vi "Lockin_sweep.vi"(8 "error in (no error)":errorcluster, 10 "Configure Sweep":T2 {"Channels"."Table" format="%#_1f"; "Channels"."Channel" min=1 max=128; "Channels"."Start" format="%#_6p"; "Channels"."End" format="%#_6p"}, 11 "Transport":refnum<class "SMO.Transport.lvclass">) -> (0 "error out":errorcluster, 3 "Transport out":refnum<class "SMO.Transport.lvclass">)   [LabVIEW 2019, in "SMO.Transport.lvclass"]
uses:
  SMO.Transport.lvclass
  <userlib>/LevyLab/Instrument Framework/Instrument Types/Cryostat/Instrument.Cryostat.lvclass
  Control Experiment/Control Experiment.lvclass
  <userlib>/LevyLab/Krohn Hite 7008/Instrument.KH7008.lvclass
  <userlib>/LevyLab/Lockin-Multichannel/Instrument.Lockin/Instrument.Lockin.lvclass
  Control Experiment/Typedefs/Instruments--cluster.ctl
  <userlib>/LevyLab/Instrument Framework/Instrument Types/VSource/Instrument.VSource.lvclass
  <userlib>/LevyLab/Instrument Framework/Instrument Types/VNA/Instrument.VNA.lvclass
  <userlib>/LevyLab/Instrument Framework/Instrument Types/Strain/Instrument.Strain.lvclass
  <userlib>/LevyLab/Instrument Framework/Instrument Types/CBridge/Instrument.CBridge.lvclass
  <userlib>/LevyLab/Lockin-Multichannel/Instrument.DAQ/Typedefs/Sweep.Configuration--Cluster.ctl
  <userlib>/LevyLab/Lockin-Multichannel/Instrument.DAQ/Instrument.DAQ.lvclass
  <userlib>/LevyLab/Lockin-Multichannel/Instrument.DAQ/Typedefs/Set State-enum.ctl
  <userlib>/_OpenG.lib/array/array.llb/Index 1D Array Elements (Variant)__ogtk.vi
  <userlib>/LevyLab/Lockin-Multichannel/Instrument.Lockin/Typedefs/Results Type--Enum.ctl
  <userlib>/LevyLab/Instrument Framework/Instrument Types/Delay Line/Instrument.DelayLine.lvclass
  <userlib>/LevyLab/Lockin-Multichannel/Instrument.DAQ/Typedefs/Sweep.Pattern--Enum.ctl
  <userlib>/LevyLab/Lockin-Multichannel/Instrument.DAQ/Typedefs/Sweep.Channel--Cluster.ctl
  <userlib>/LevyLab/Lockin-Multichannel/Instrument.DAQ/Typedefs/Sweep.Channel--Cluster--Array.ctl
  SMO.Control Experiment/SMO.Control Experiment.lvclass
  C:/Program Files (x86)/National Instruments/LabVIEW 2019/user.lib/LevyLab/Instrument Framework/SMOs/Instrument/Instrument.lvclass
  C:/Program Files (x86)/National Instruments/LabVIEW 2019/vi.lib/JKI/JKI SMO/SMO/SMO.lvclass
panel:
  in  "Tab Control":T1(tab)
  out "elapsed time (s)":u32=231
  in  "Experiment Comments":string="sweep inplane y gates in differential mode, 110Mohm resistor on each\nlead 3: +X: 0 V\nlead 15: -X: 0V\nlead 8: +Y: -10V to 10V to -10V to 10V...\nlead 21: -Y: 10V to -10V to 10V to -10V..\n\nInital wait: 2s+ 2s\nSweep Time: 90s+90s\n\nstripe device\nI+: 11,12, current mode, 5k resistor on each, 1000x gain\nlead 12: Vac: 125uV, 7Hz. Vdc=0mV\ndV: KH channel 16: 11-12, differential voltage meas, 10x gain \n\nhash device\nI+: 16,27, current mode, 5k resistor on each, 1000x gain\nlead 16: Vac: 5mV, 7Hz. Vdc=0mV\nV+/V-: 17/20, voltage meas, 10x gain \nKH 5: 17-20, volt. meas., 10x gain\n\n\nlead 26: Vbg: 0V, 1Gohm resistor\nB: -18T to 18T @0.033T/min\n"
  in  "Experiment Folder":string="23-Lockinsweep_ygates_-18_18"
  out "T (mK)":dbl=0.001
  out "Field (T)":dbl=0.0037 format="%#_13g"
  out "time b/w points (ms)":u32=1037
  in  "stop":bool
  out "X Lockins":cluster{dbl[], dbl[]}[](graph)
  out "Y Lockins":cluster{dbl[], dbl[]}[](graph)
  out "G4T":cluster{dbl[], dbl[]}[](graph)
  out "AI Waveform":waveform(dbl)[](graph)
  out "AO Waveform":waveform(dbl)[](graph)
  in  "AO indices":i32[](array[numeric])
  in  "AI indices":i32[](array[numeric])
  out "2Term":T6(graph)
  out "4Term":cluster{dbl[], dbl[]}[](graph)
  # "VI description:\nThis VI uses the Lockin Sweep Method. That is, you tell the lockin to sweep from Start to End in a certain amount of time. The lockin will run independently while it executes the sweep. While the lockin is sweeping, this VI will poll the lockin once per second to get a snapshot of current results and the sweep status (sweeping or not sweeping). When the lockin is finished sweeping this VI will ask for the final sweep results and save them."
  # "*** These controls are only read if this VI is the top level. If is is called from Sweep Control then the folder and comments come from Sweep Control.vi ***"
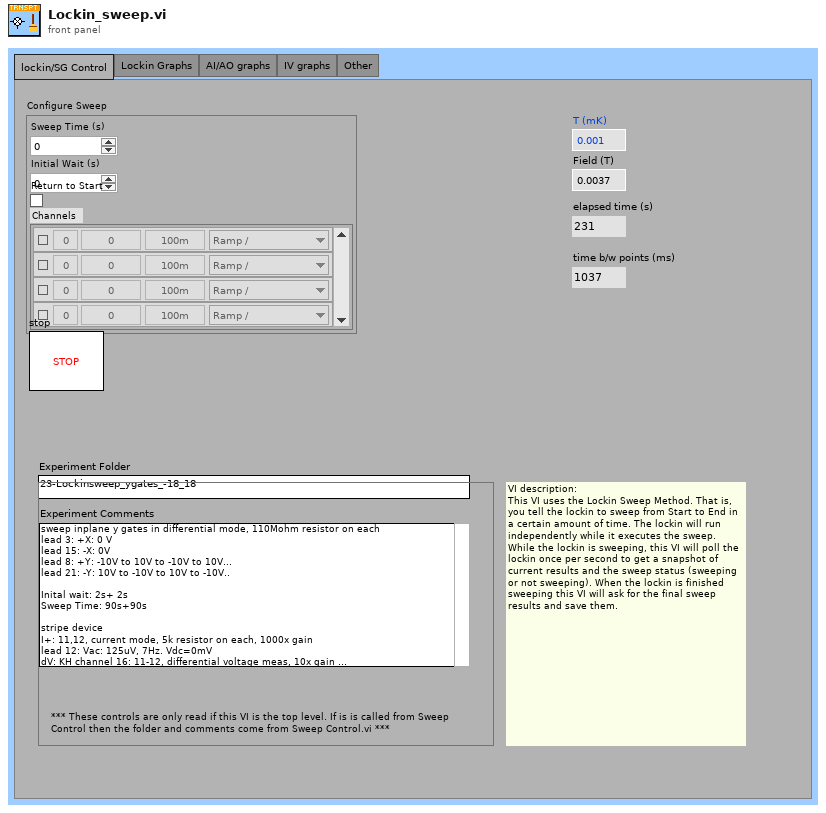
[diagram p1: front panel]
types:
  T1 = enum32{"lockin/SG Control", "Lockin Graphs", "AI/AO graphs", "IV graphs", "Other"}
  T2 = typedef "Instrument.DAQ.lvclass/Sweep.Configuration--Cluster.ctl" = cluster{"Sweep Time (s)":dbl, "Initial Wait (s)":dbl, "Return to Start":bool, "Channels":T3}
  T3 = typedef "Instrument.DAQ.lvclass/Sweep.Channel--Cluster--Array.ctl" = T4[]
  T4 = typedef "Instrument.DAQ.lvclass/Sweep.Channel--Cluster.ctl" = cluster{"Enable?":bool, "Channel":u16, "Start":dbl, "End":dbl, "Pattern":T5, "Table":dbl[]}
  T5 = typedef "Instrument.DAQ.lvclass/Sweep.Pattern--Enum.ctl" = enum16{"Ramp /", "Ramp /\\", "Smooth Ramp _/", "Smooth Ramp _/\\_", "Table"}
  T6 = cluster{"Decimated and Filtered Array":dbl[], "Decimated and Filtered Array":dbl[]}[]
  T7 = enum32{"Invalid", "Standard", "Closed", "Hidden", "Minimized", "Maximized"}
  T8 = enum32{"invalid app kind", "Development System", "Run Time System", "Student Edition", "Embedded LabVIEW", "Evaluation", "Custom"}
  T9 = typedef "Instrument.Lockin.lvclass/Results Type--Enum.ctl" = enum16{"X", "Y", "R", "Theta", "Mean"}
  T10 = typedef "Lockin.DAQ.lvclass/State-enum.ctl" = enum16{"idle", "created", "started", "stopped", "sweeping"}
  T11 = typedef "Control Experiment.lvclass/Instruments--cluster.ctl" = cluster{"KH7008":refnum<class "Instrument.KH7008.lvclass">[], "Lockin":refnum<class "Instrument.Lockin.lvclass">, "Temperature":refnum<class "Instrument.Cryostat.lvclass">, "Magnet":refnum<class "Instrument.Cryostat.lvclass">, "Rotator":refnum<class "Instrument.Cryostat.lvclass">, "Level":refnum<class "Instrument.Cryostat.lvclass">, "Capacitance Bridge":refnum<class "Instrument.CBridge.lvclass">, "Delay Line":refnum<class "Instrument.DelayLine.lvclass">, "Strain Cell":refnum<class "Instrument.Strain.lvclass">, "VNA":refnum<class "Instrument.VNA.lvclass">, "Voltage Source":refnum<class "Instrument.VSource.lvclass">}
  T12 = cluster{"Core":cluster{"Current VI Reference":refnum<vi>, "Close Panel on Exit?":bool}, "Transport":refnum<class "SMO.Transport.lvclass">, "Control Experiment":refnum<class "SMO.Control Experiment.lvclass">, "Instruments":T11, "Time":dbl, "Temperature":dbl, "Magnet":dbl, "Results (Dictionary)":cluster{"key":string, "value":dbl}[], "Sweep Value":dbl, "ms [0]":u32, "ms [i]":u32, "Execution:State":enum32{"Bad", "Idle", "Run top level", "Running"}, "AO Waveforrm":waveform(dbl)[], "AI Waveform":waveform(dbl)[], "Sweep_AO":waveform(dbl)[], "Sweep_AI":waveform(dbl)[]}
  T13 = enum32{"Bad", "Idle", "Run top level", "Running"}
  T14 = cluster{"Current VI Reference":refnum<vi>, "Close Panel on Exit?":bool}
  T15 = cluster{"I-":i32, "I+":i32, "V1-":i32, "V1+":i32, "I2-":i32, "I2+":i32, "V2-":i32, "V2+":i32}
  T16 = typedef "Instrument.DAQ.lvclass/Get State-enum.ctl" = enum16{"idle", "created", "started", "stopped", "sweeping"}
  T17 = typedef "Instrument.DAQ.lvclass/AO.Channel--Cluster--Array.ctl" = T18[]
  T18 = typedef "Instrument.DAQ.lvclass/AO.Channel--Cluster.ctl" = cluster{"Enable?":bool, "Channel":i32, "Amplitude":dbl, "Offset":dbl, "Frequency":dbl, "Phase":dbl, "Function":T19, "Sweeping?":bool}
  T19 = typedef "Instrument.DAQ.lvclass/AO.Channel.Function--Enum.ctl" = enum16{"Sine", "Triangle", "Square"}
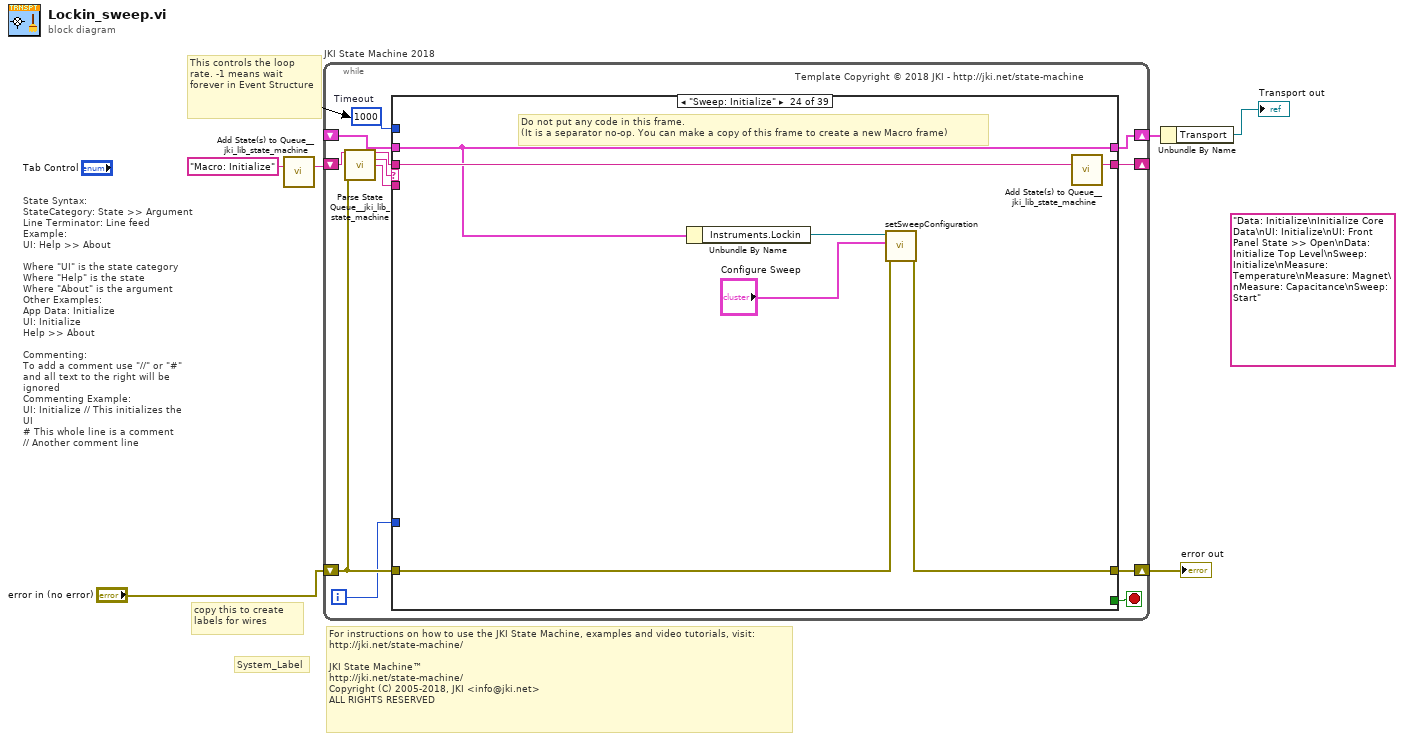
[diagram p0: block diagram]
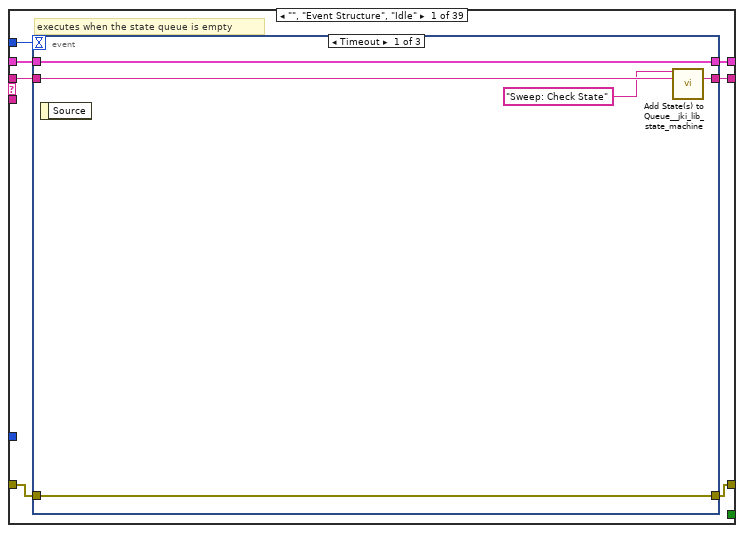
[diagram p2: hidden frame]
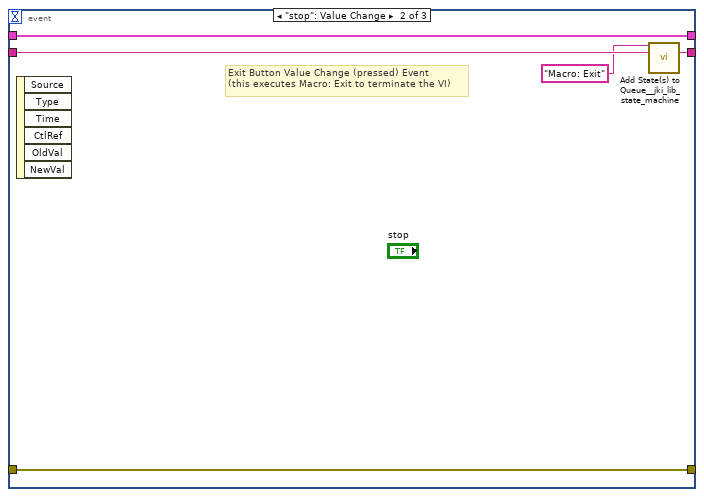
[diagram p3: hidden frame]
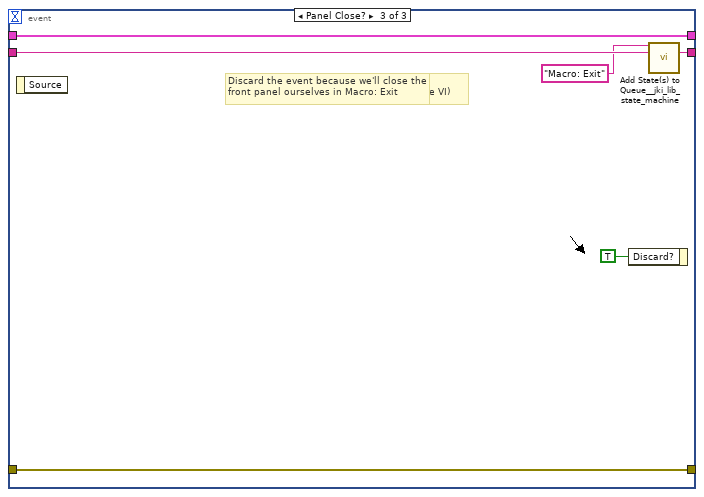
[diagram p4: hidden frame]
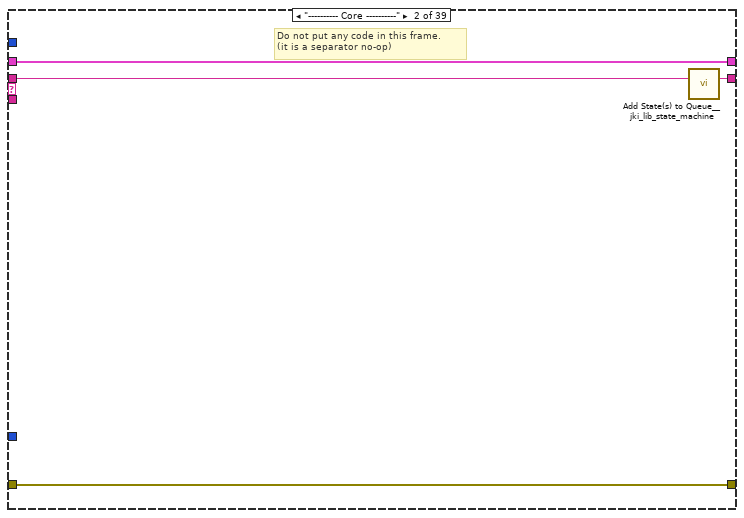
[diagram p5: hidden frame]
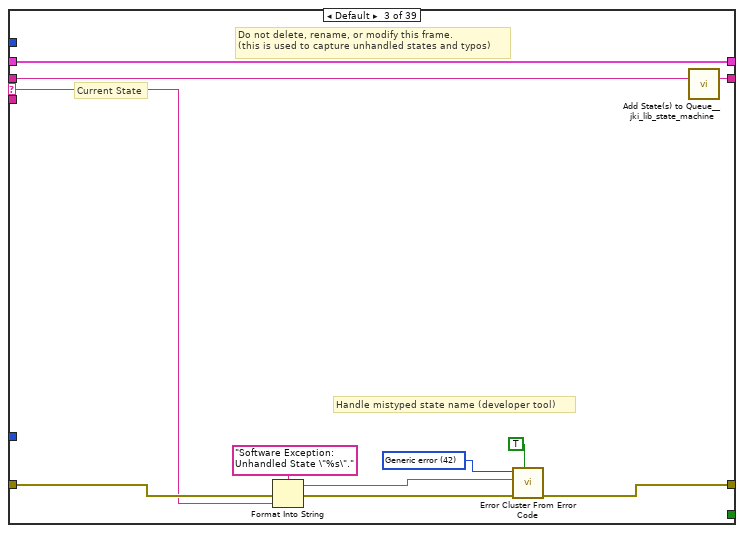
[diagram p6: hidden frame]
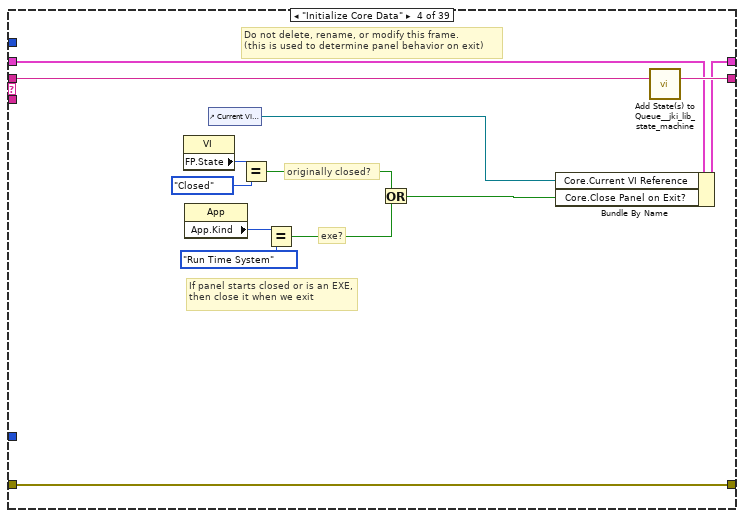
[diagram p7: hidden frame]
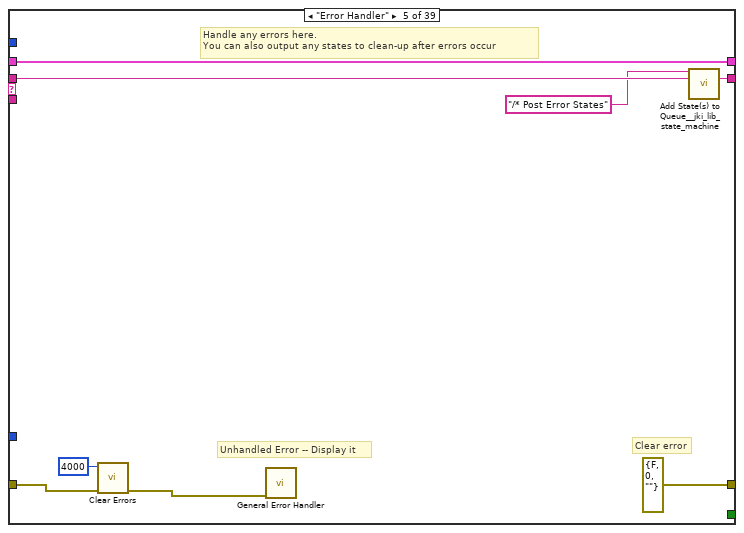
[diagram p8: hidden frame]
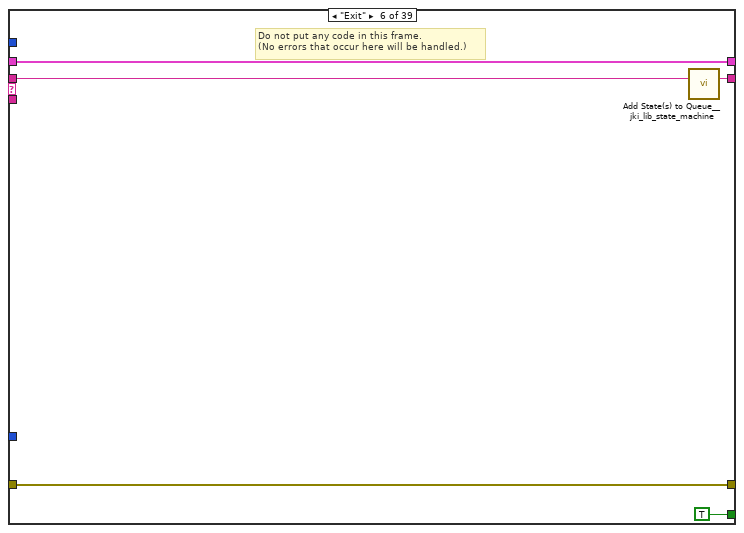
[diagram p9: hidden frame]
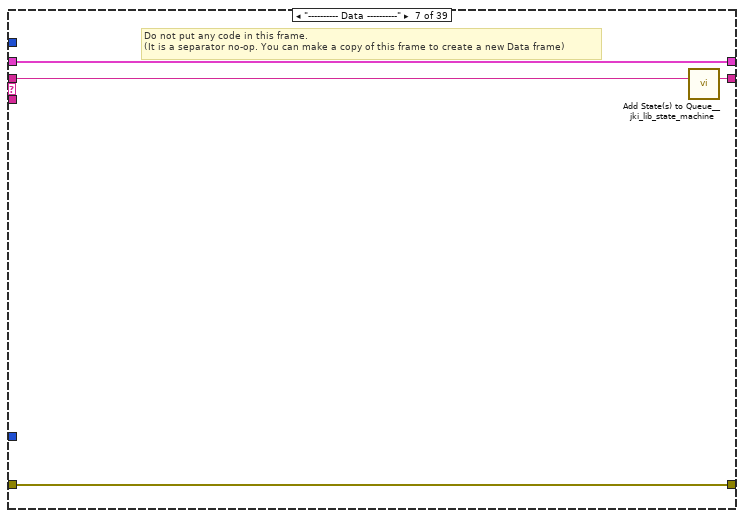
[diagram p10: hidden frame]
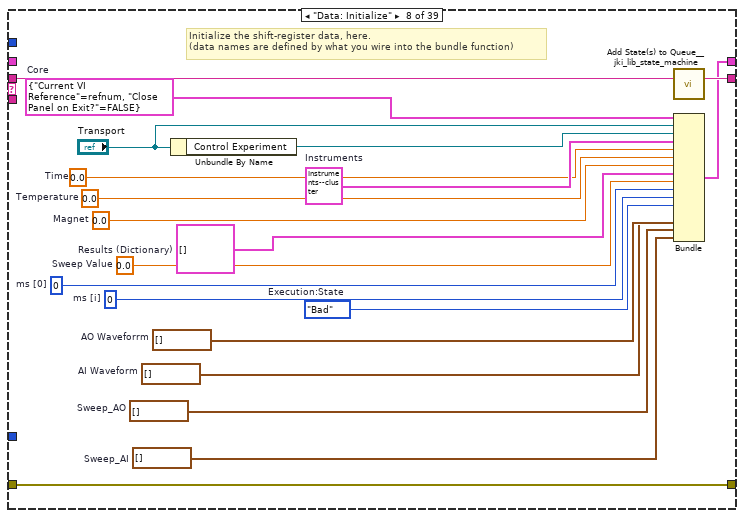
[diagram p11: hidden frame]
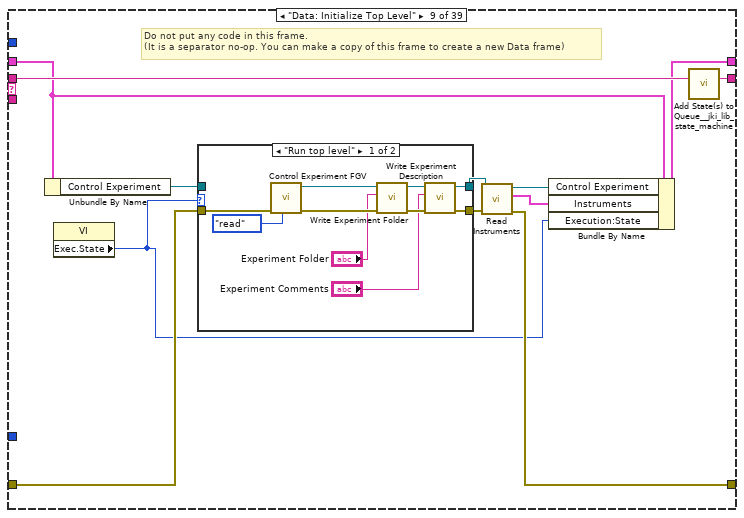
[diagram p12: hidden frame]
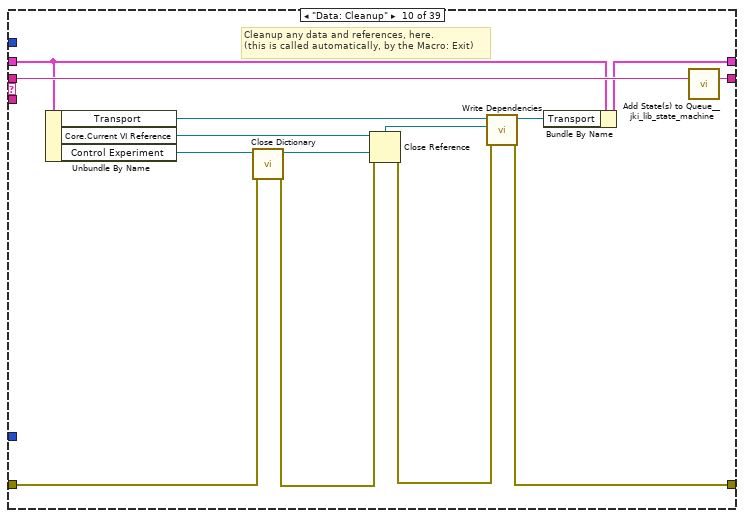
[diagram p14: hidden frame]
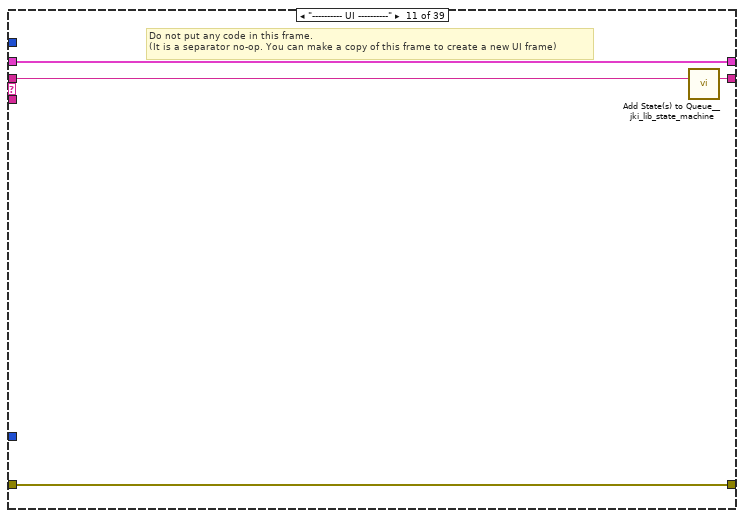
[diagram p15: hidden frame]
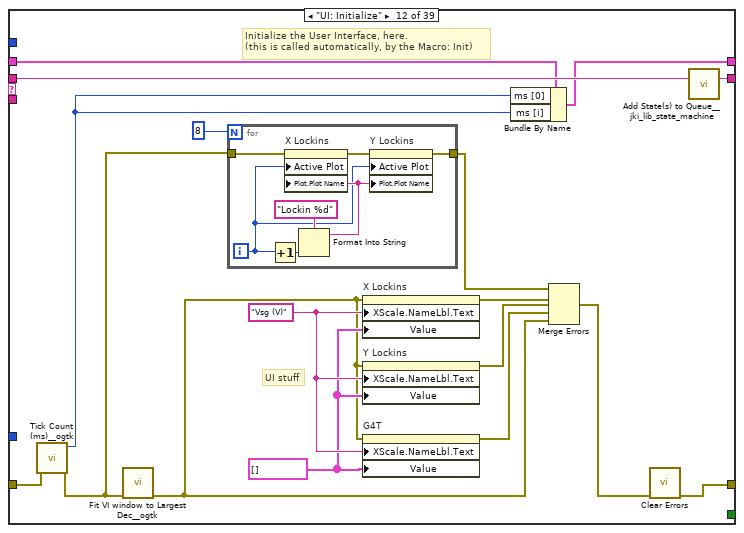
[diagram p16: hidden frame]
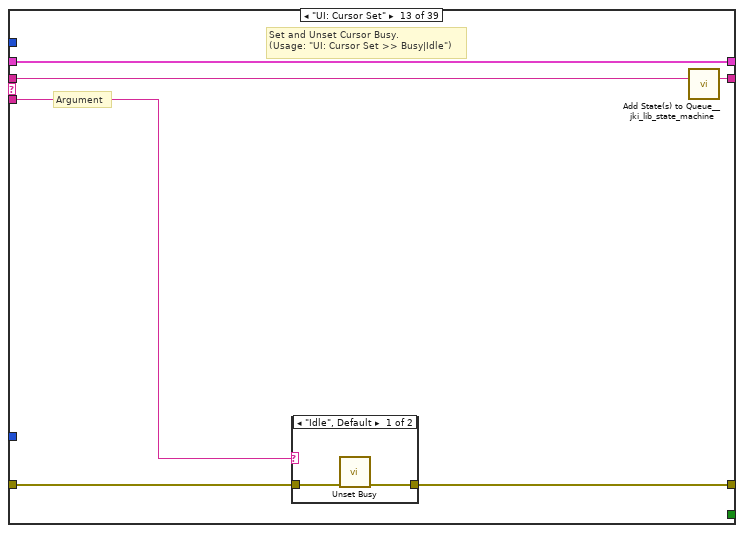
[diagram p17: hidden frame]
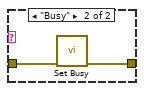
[diagram p18: hidden frame]
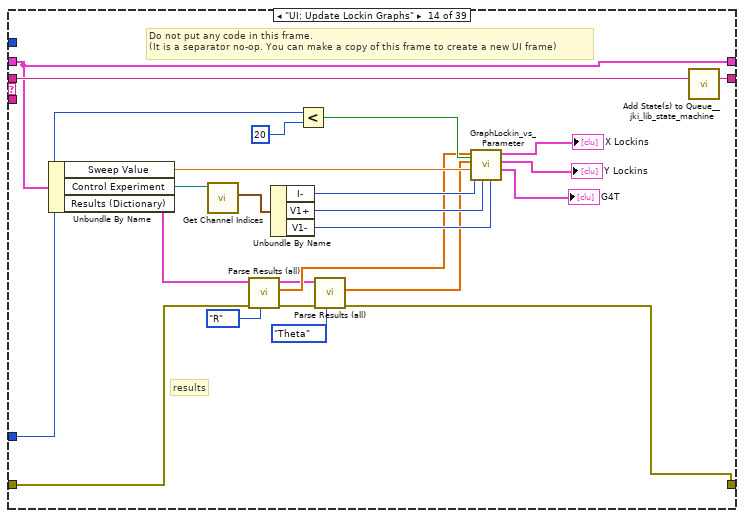
[diagram p19: hidden frame]
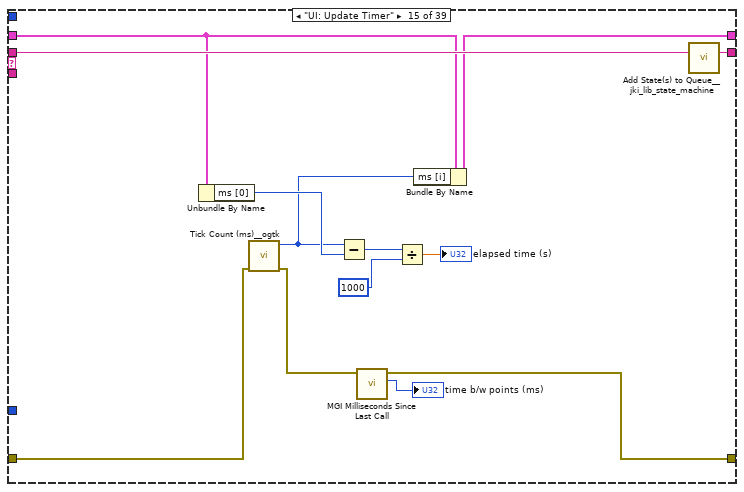
[diagram p20: hidden frame]
diagram:
  (unwired) "Data: Initialize\nInitialize Core Data\nUI: Initialize\nUI: Front Panel State >> Open\nData: Initialize Top Level\nSweep: Initialize\nMeasure: Temperature\nMeasure: Magnet\nMeasure: Capacitance\nSweep: Start"
  # "For instructions on how to use the JKI State Machine, examples and video tutorials, visit:\nhttp://jki.net/state-machine/\n\nJKI State Machine™\nhttp://jki.net/state-machine/\nCopyright (C) 2005-2018, JKI <info@jki.net>\nALL RIGHTS RESERVED"
  # "State Syntax:\nStateCategory: State >> Argument\nLine Terminator: Line feed\nExample:\nUI: Help >> About\n\nWhere \"UI\" is the state category\nWhere \"Help\" is the state\nWhere \"About\" is the argument\nOther Examples:\nApp Data: Initialize\nUI: Initialize\nHelp >> About\n\nCommenting:\nTo add a comment use \"//\" or \"#\" and all text to the right will be ignored\nCommenting Example:\nUI: Initialize // This initializes the UI\n# This whole line is a comment\n// Another comment line"
  # "copy this to create labels for wires"
  # "This controls the loop rate. -1 means wait forever in Event Structure"
  # "System_Label"
  n1 = call <vilib>:"Add State(s) to Queue__jki_lib_state_machine.vi"("State(s) in (\"\")"="Macro: Initialize") -> ("States Out"=w6:string)  [unwired: 14 in]
  n2 = while "JKI State Machine 2018" {
    shift-right: [w11] -> w4
    shift-left: _ -> [w10]
    shift-right: [w14] -> w2
    shift-left: "error in (no error)" -> [w8]
    shift-right: [w13] -> _
    shift-left: w6 -> [w15]
    i -> [w7]
    stop <- w12 stop-if-true
    w9 = 1000  # Timeout
    # "Template Copyright © 2018 JKI - http://jki.net/state-machine"
    n3 = call <vilib>:"Parse State Queue__jki_lib_state_machine.vi"("State Queue"=w15, "Error In (no error)"=w8) -> ("Remaining States"=w17:string, "Current State"=w18:string, "Arguments"=w16:string)  [unwired: 11 in]
    n4 = case shown="\"Sweep: Initialize\"" w18 {
      selector: w18 -> [_ _ w46 _ _ _ _ _ _ _ _ _ _ _ _ _ _ _ _ _ _ _ _ _ _ _ _ _ _ _ _ _ _ _ _ _ _ _ _]
      tunnel: w17 -> [w25 w45 w50 w69 w77 w82 w86 w106 w118 w143 w147 w164 w177 w205 w218 w232 w263 w270 w339 w344 w349 w359 w363 w370 w378 w393 w401 w407 w411 w415 w426 w439 w452 w464 w486 w490 w494 w527 w546]
      tunnel: w16 -> [_ _ _ _ _ _ _ _ _ _ _ _ w172 _ _ _ _ w264 _ _ _ _ _ _ _ _ _ _ _ _ _ _ _ _ _ _ _ _ _]
      tunnel: w10 -> [w23 w42 w48 w62 w74 w80 w83 _ w109 w131 w144 w152 w175 w202 w213 w222 w242 w266 w336 w342 w345 w356 w360 w365 w376 w391 w399 w404 w409 w412 w422 w435 w450 w453 w465 w487 w491 w516 w543]
      tunnel: [w22 w43 w52 w66 errorcluster {"status"=FALSE, "code"=0, "source"=""} ("error out") w79 w84 w103 w110 w133 w145 w156 w173 w182 w207 w230 w240 w267 w337 w340 w347 w357 w361 w366 w371 w388 w396 w405 w408 w413 w416 w428 w446 w459 w484 w488 w492 w519 w541] -> w14
      tunnel: w8 -> [w21 w43 w51 w66 w71 w79 w84 w103 w111 w139 w145 w154 w174 w184 w215 w230 w241 w268 w337 w340 w347 w357 w361 w367 w374 w389 w397 w405 w408 w413 w417 w436 w443 w457 w482 w488 w492 w498 w542]
      tunnel: [w24 w44 w49 w68 w76 w81 w85 w105 w117 w142 w146 w163 w176 w204 w217 w231 w262 w269 w338 w343 w348 w358 w362 w369 w377 w392 w400 w406 w410 w414 w425 w438 w451 w463 w485 w489 w493 w526 w545] -> w13
      tunnel: [_ _ _ _ _ TRUE _ _ _ _ _ _ _ _ _ _ _ _ _ _ _ _ _ _ _ _ _ _ _ _ _ _ _ _ _ _ _ _ _] -> w12
      tunnel: [w20 w42 w48 w67 w74 w80 w83 w104 w108 w135 w144 w151 w175 w202 w212 w221 w242 w266 w336 w342 w345 w356 w360 w365 w376 w391 w399 w404 w409 w412 w423 w434 w449 w462 w466 w487 w491 w515 w543] -> w11
      tunnel: w9 -> [w19 _ _ _ _ _ _ _ _ _ _ _ _ _ _ _ _ _ _ _ _ _ _ _ _ _ _ _ _ _ _ _ _ _ _ _ _ _ _]
      tunnel: w7 -> [_ _ _ _ _ _ _ _ _ _ _ _ _ w193 _ _ _ _ _ _ _ _ _ _ _ _ _ _ _ _ _ _ _ _ _ _ _ _ _]
      frame "", "Event Structure", "Idle" {
        # "executes when the state queue is empty"
        n5 = event shown="[0] Timeout" {
          selector: _ -> [_ _ _]
          dyn-events: _ -> [_ _ _]
          timeout: w19 -> [_ _ _]
          tunnel: w25 -> [w30 w35 w41]
          tunnel: [w29 w34 w40] -> w24
          tunnel: w23 -> [w27 w32 w38]
          tunnel: [w28 w33 w39] -> w22
          tunnel: w21 -> [w28 w33 w39]
          tunnel: [w27 w32 w38] -> w20
          event Timeout {
            n6 = event-data() -> ()  [unwired: 1 in, 1 out]
            n7 = call <vilib>:"Add State(s) to Queue__jki_lib_state_machine.vi"("State(s) in Front (\"\")"="Sweep: Check State" ("State(s) in Front (\"\")"), "State(s) in (\"\")"=w30) -> ("States Out"=w29:string)  [unwired: 13 in]
          }
          event "stop": Value Change {
            # "Exit Button Value Change (pressed) Event\n(this executes Macro: Exit to terminate the VI)"
            n8 = event-data() -> ()  [unwired: 1 in, 6 out]
            n9 = call <vilib>:"Add State(s) to Queue__jki_lib_state_machine.vi"("State(s) in Front (\"\")"="Macro: Exit", "State(s) in (\"\")"=w35) -> ("States Out"=w34:string)  [unwired: 13 in]
          }
          event Panel Close? {
            # "Discard the event because we'll close the front panel ourselves in Macro: Exit"
            # "Close Panel button (pressed) Event\n(this executes Macro: Exit to terminate the VI)"
            n10 = event-data() -> ()  [unwired: 1 in, 1 out]
            n11 = event-data("Discard?"=TRUE) -> ()  [unwired: 1 in, 1 out]
            n12 = call <vilib>:"Add State(s) to Queue__jki_lib_state_machine.vi"("State(s) in Front (\"\")"="Macro: Exit", "State(s) in (\"\")"=w41) -> ("States Out"=w40:string)  [unwired: 13 in]
          }
        }
      }
      frame "---------- Core ----------" {
        # "Do not put any code in this frame.\n(it is a separator no-op)"
        n13 = call <vilib>:"Add State(s) to Queue__jki_lib_state_machine.vi"("State(s) in (\"\")"=w45) -> ("States Out"=w44:string)  [unwired: 14 in]
      }
      frame Default {
        w55 = 42 items=["No error", "Argument error", "Memory is full", "Out of zone", "End of file", "File already open", "Generic file I/O error", "File not found", "File permission error", "Disk is full", "Duplicate path", "Too many files open", "System feature not enabled", "Resource file not found", "Cannot add resource", "Resource not found", "Image not found", "Image memory error", "Pen does not exist", "Config type invalid", "Config token not found", "Config parse error", "Config memory error", "Bad external code format", "Bad external code offset", "External code not present", "Null window", "Destroy window error", "Null menu", "Print aborted", "Bad print record", "Print driver error", "Windows error during printing", "Memory error during printing", "Print dialog error", "Generic print error", "Invalid device refnum", "Device not found", "Device parameter error", "Device unit error", "Cannot open device", "Device call aborted", "Generic error", "Cancelled by user", "Object ID too low", "Object ID too high", "Object not in heap", "Unknown heap", "Unknown object (invalid DefProc)", "Unknown object (DefProc not in table)", "Message out of range", "Invalid (null) method", "Unknown message", "Manager call not supported", "Bad address", "Network operation in progress", "Network operation timed out", "Connection is busy", "Network attribute not supported", "Network error", "Address in use", "System out of memory", "Connection aborted", "Connection refused", "Not connected", "Already connected", "Connection closed", "Initialization error (interapplication manager)", "Bad occurrence", "Wait on unbound occurrence handler", "Occurrence queue overflow", "Datalog type conflict", "Unused", "Unrecognized type (interapplication manager)", "Memory corrupt", "Failed to make temporary DLL", "Old CIN version", "Drag socket not found", "Failed to load drop-object", "Failed to register OLE object", "Failed to release OLE object", "Format specifier type mismatch", "Unknown format specifier", "Too few format specifiers", "Too many format specifiers", "Scan failed", "Newer CIN version", "Error converting to variant", "Runtime menu error", "Password tampered", "Variant attribute not found", "Incompatible variant data type", "Event data is not available", "Event Store is not present", "Occurrence is not found", "Event Queue is not created", "Event info is not available", "Refnum passed is NULL", "Error retrieving Class GUID", "Error retrieving CoClass GUID", "Error retrieving TypeLib GUID.", "Bad built application magic bytes.", "Specific driver is different from the specific driver associated with the Logical Name.", "There is no session opened to the class driver.", "Max Error", "MAX - Error with config objects", "MAX - Error loading configuration", "MAX - Group not supported"]
        # "Current State"
        # "Do not delete, rename, or modify this frame.\n(this is used to capture unhandled states and typos)"
        # "Handle mistyped state name (developer tool)"
        n14 = Format Into String(format string="Software Exception: Unhandled State \"%s\"." ("message"), error in=w51, w46) -> (resulting string=w54:string, error out=w53:errorcluster)  [unwired: 1 in]
        n15 = call <vilib>:"Error Cluster From Error Code.vi"("show call chain? (False)"=TRUE, "error in (no error)"=w53, "error message (\"\")"=w54, "error code (0)"=w55) -> ("error out"=w52:errorcluster)  [unwired: 5 in]
        n16 = call <vilib>:"Add State(s) to Queue__jki_lib_state_machine.vi"("State(s) in (\"\")"=w50) -> ("States Out"=w49:string)  [unwired: 14 in]
      }
      frame "Initialize Core Data" {
        # "Do not delete, rename, or modify this frame.\n(this is used to determine panel behavior on exit)"
        # "originally closed?"
        # "exe?"
        # "If panel starts closed or is an EXE, then close it when we exit"
        n17 = property class="VI"() -> ("FP.State"=w59:T7)  [unwired: 2 in, 2 out]
        n18 = property class="App"() -> ("App.Kind"=w65:T8)  [unwired: 2 in, 2 out]
        n19 = control-ref of="Current VI Reference"() -> (w60:refnum<vi>)
        n20 = Equal?(x=w59, y=T7."Closed" ("Front Panel Window:State")) -> (x = y?=w57:bool)
        n21 = Equal?(x=w65, y=T8."Run Time System" ("Application:Kind")) -> (x = y?=w63:bool)
        n22 = Or(x=w57, y=w63) -> (x .or. y?=w61:bool)
        n23 = Bundle By Name(cluster=w62, "Core.Current VI Reference"=w60, "Core.Close Panel on Exit?"=w61) -> (w67:T12)
        n24 = call <vilib>:"Add State(s) to Queue__jki_lib_state_machine.vi"("State(s) in (\"\")"=w69) -> ("States Out"=w68:string)  [unwired: 14 in]
      }
      frame "Error Handler" {
        # "Unhandled Error -- Display it"
        # "Handle any errors here.\nYou can also output any states to clean-up after errors occur"
        # "Clear error"
        n25 = call <vilib>:"Clear Errors.vi"("error in (no error)"=w71, "specific error code to clear (0: all)"=4000) -> ("error out"=w70:errorcluster)  [unwired: 4 in, 1 out]
        n26 = call <vilib>:"General Error Handler.vi"("error in (no error)"=w70) -> ()  [unwired: 10 in, 5 out]
        n27 = call <vilib>:"Add State(s) to Queue__jki_lib_state_machine.vi"("State(s) in Front (\"\")"="/* Post Error States", "State(s) in (\"\")"=w77) -> ("States Out"=w76:string)  [unwired: 13 in]
      }
      frame "Exit" {
        # "Do not put any code in this frame.\n(No errors that occur here will be handled.)"
        n28 = call <vilib>:"Add State(s) to Queue__jki_lib_state_machine.vi"("State(s) in (\"\")"=w82) -> ("States Out"=w81:string)  [unwired: 14 in]
      }
      frame "---------- Data ----------" {
        # "Do not put any code in this frame.\n(It is a separator no-op. You can make a copy of this frame to create a new Data frame)"
        n29 = call <vilib>:"Add State(s) to Queue__jki_lib_state_machine.vi"("State(s) in (\"\")"=w86) -> ("States Out"=w85:string)  [unwired: 14 in]
      }
      frame "Data: Initialize" {
        w87 = cluster{"key":string, "value":dbl}[] []  # Results (Dictionary)
        w89 = waveform(dbl)[] []  # Sweep_AO
        w88 = waveform(dbl)[] []  # Sweep_AI
        w90 = waveform(dbl)[] []  # AI Waveform
        w91 = waveform(dbl)[] []  # AO Waveforrm
        w92 = T13."Bad"  # Execution:State
        w93 = 0.0  # Sweep Value
        w95 = u32 0  # ms [i]
        w96 = u32 0  # ms [0]
        w98 = 0.0  # Time
        w99 = 0.0  # Magnet
        w97 = 0.0  # Temperature
        w100 = T11 {"KH7008"=[], "Lockin"=refnum, "Temperature"=refnum, "Magnet"=refnum, "Rotator"=refnum, "Level"=refnum, "Capacitance Bridge"=refnum, "Delay Line"=refnum, "Strain Cell"=refnum, "VNA"=refnum, "Voltage Source"=refnum}  # Instruments
        w102 = T14 {"Current VI Reference"=refnum, "Close Panel on Exit?"=FALSE}  # Core
        # "Initialize the shift-register data, here.\n(data names are defined by what you wire into the bundle function)"
        n30 = Unbundle By Name("Transport") -> ("Control Experiment"=w94:refnum<class "SMO.Control Experiment.lvclass">)
        n31 = call <vilib>:"Add State(s) to Queue__jki_lib_state_machine.vi"("State(s) in (\"\")"=w106) -> ("States Out"=w105:string)  [unwired: 14 in]
        n32 = Bundle("Core"=w102, "Transport"="Transport", "Control Experiment"=w94, "Instruments"=w100, "Time"=w98, "Temperature"=w97, "Magnet"=w99, "Results (Dictionary)"=w87, "Sweep Value"=w93, "ms [0]"=w96, "ms [i]"=w95, "Execution:State"=w92, "AO Waveforrm"=w91, "AI Waveform"=w90, "Sweep_AO"=w89, "Sweep_AI"=w88) -> (w104:T12)  [unwired: 1 in]
      }
      frame "Data: Initialize Top Level" {
        # "Do not put any code in this frame.\n(It is a separator no-op. You can make a copy of this frame to create a new Data frame)"
        n33 = Unbundle By Name(w109) -> ("Control Experiment"=w112:refnum<class "SMO.Control Experiment.lvclass">)
        n34 = property class="VI"() -> ("Exec.State"=w107:T13)  [unwired: 2 in, 2 out]
        n35 = case shown="\"Run top level\"" w107 {
          tunnel: w111 -> [w128 w129]
          tunnel: [w123 w129] -> w113
          tunnel: [w122 w130] -> w114
          tunnel: w112 -> [_ w130]
          frame "Run top level" {
            n36 = call "Control Experiment FGV.vi"("Function"=enum16{"read", "write"}."read", "error in (no error)"=w128) -> ("error out"=w126:errorcluster, "Control Experiment.lvclass out"=w127:refnum<class "Control Experiment.lvclass">)  [unwired: 8 in]
            n37 = call "Write Experiment Folder.vi"("error in (no error)"=w126, "Experiment Folder"="Experiment Folder", "Control Experiment in"=w127) -> ("error out"=w124:errorcluster, "Control Experiment out"=w125:refnum<class "Control Experiment.lvclass">)  [unwired: 7 in]
            n38 = call "Write Experiment Description.vi"("error in (no error)"=w124, "Experiment Description"="Experiment Comments", "Control Experiment in"=w125) -> ("error out"=w123:errorcluster, "Control Experiment out"=w122:refnum<class "Control Experiment.lvclass">)  [unwired: 7 in]
          }
          frame "Running", Default {
          }
        }
        n39 = call "Read Instruments.vi"("error in (no error)"=w113, "Control Experiment in"=w114) -> ("error out"=w110:errorcluster, "Instruments"=w116:T11, "Control Experiment out"=w115:refnum<class "Control Experiment.lvclass">)  [unwired: 7 in]
        n40 = Bundle By Name(cluster=w109, "Control Experiment"=w115, "Instruments"=w116, "Execution:State"=w107) -> (w108:T12)
        n41 = call <vilib>:"Add State(s) to Queue__jki_lib_state_machine.vi"("State(s) in (\"\")"=w118) -> ("States Out"=w117:string)  [unwired: 14 in]
      }
      frame "Data: Cleanup" {
        # "Cleanup any data and references, here.\n(this is called automatically, by the Macro: Exit)"
        n42 = Unbundle By Name(w131) -> ("Transport"=w136:refnum<class "SMO.Transport.lvclass">, "Core.Current VI Reference"=w141:refnum<vi>, "Control Experiment"=w140:refnum<class "SMO.Control Experiment.lvclass">)
        n43 = call "Close Dictionary.vi"("error in (no error)"=w139, "Control Experiment in"=w140) -> ("error out"=w138:errorcluster, "Control Experiment out"=w132:refnum<class "Control Experiment.lvclass">)  [unwired: 8 in]
        n44 = Close Reference(reference=w141, error in (no error)=w138) -> (error out=w134:errorcluster)
        n45 = call "Write Dependencies.vi"("error in (no error)"=w134, "Control Experiment"=w132, "Transport in"=w136) -> ("error out"=w133:errorcluster, "Transport out"=w137:refnum<class "SMO.Transport.lvclass">)  [unwired: 7 in]
        n46 = Bundle By Name(cluster=w131, "Transport"=w137) -> (w135:T12)
        n47 = call <vilib>:"Add State(s) to Queue__jki_lib_state_machine.vi"("State(s) in (\"\")"=w143) -> ("States Out"=w142:string)  [unwired: 14 in]
      }
      frame "---------- UI ----------" {
        # "Do not put any code in this frame.\n(It is a separator no-op. You can make a copy of this frame to create a new UI frame)"
        n48 = call <vilib>:"Add State(s) to Queue__jki_lib_state_machine.vi"("State(s) in (\"\")"=w147) -> ("States Out"=w146:string)  [unwired: 14 in]
      }
      frame "UI: Initialize" {
        w149 = cluster{dbl[], dbl[]}[] [] ("G4T")
        w158 = "Vsg (V)" ("string")
        # "UI stuff"
        # "Initialize the User Interface, here.\n(this is called automatically, by the Macro: Init)"
        n49 = call <userlib>:"Tick Count (ms)__ogtk.vi"("error in (no error)"=w154) -> ("error out"=w153:errorcluster, "millisecond timer value"=w150:u32)  [unwired: 9 in]
        n50 = call <userlib>:"Fit VI window to Largest Dec__ogtk.vi"("error in (no error)"=w153) -> ("error out"=w148:errorcluster)  [unwired: 5 in, 1 out]
        n51 = for {
          N: 8 -> [_]
          tunnel: [w165] -> w159
          tunnel: w153 -> [w170]
          i -> [w168]
          n52 = Increment(x=w168) -> (x+1=w166:i32)
          n53 = Format Into String(format string="Lockin %d", w166) -> (resulting string=w169:string)  [unwired: 2 in, 1 out]
          n54 = property on="X Lockins" class="XYGraph (strict)"(error in=w170, "Active Plot"=w168, "Plot.Plot Name"=w169) -> (error out=w167:errorcluster)  [unwired: 1 in, 1 out]
          n55 = property on="Y Lockins" class="XYGraph (strict)"(error in=w167, "Active Plot"=w168, "Plot.Plot Name"=w169) -> (error out=w165:errorcluster)  [unwired: 1 in, 1 out]
        }
        n56 = property on="X Lockins" class="XYGraph (strict)"(error in=w148, "XScale.NameLbl.Text"=w158, "Value"=w149) -> (error out=w160:errorcluster)  [unwired: 1 in, 1 out]
        n57 = property on="Y Lockins" class="XYGraph (strict)"(error in=w148, "XScale.NameLbl.Text"=w158, "Value"=w149) -> (error out=w161:errorcluster)  [unwired: 1 in, 1 out]
        n58 = property on="G4T" class="XYGraph (strict)"(error in=w148, "XScale.NameLbl.Text"=w158, "Value"=w149) -> (error out=w162:errorcluster)  [unwired: 1 in, 1 out]
        n59 = Bundle By Name(cluster=w152, "ms [0]"=w150, "ms [i]"=w150) -> (w151:T12)
        n60 = Merge Errors(w159, w160, w161, w162, w148) -> (w155:errorcluster)
        n61 = call <vilib>:"Clear Errors.vi"("error in (no error)"=w155) -> ("error out"=w156:errorcluster)  [unwired: 5 in, 1 out]
        n62 = call <vilib>:"Add State(s) to Queue__jki_lib_state_machine.vi"("State(s) in (\"\")"=w164) -> ("States Out"=w163:string)  [unwired: 14 in]
      }
      frame "UI: Cursor Set" {
        # "Argument"
        # "Set and Unset Cursor Busy.\n(Usage: \"UI: Cursor Set >> Busy|Idle\")"
        n63 = case shown="\"Idle\", Default" w172 {
          tunnel: w174 -> [w179 w181]
          tunnel: [w178 w180] -> w173
          frame "Idle", Default {
            n64 = call <vilib>:"Unset Busy.vi"("error in (no error)"=w179) -> ("error out"=w178:errorcluster)  [unwired: 10 in]
          }
          frame "Busy" {
            n65 = call <vilib>:"Set Busy.vi"("error in (no error)"=w181) -> ("error out"=w180:errorcluster)  [unwired: 9 in, 1 out]
          }
        }
        n66 = call <vilib>:"Add State(s) to Queue__jki_lib_state_machine.vi"("State(s) in (\"\")"=w177) -> ("States Out"=w176:string)  [unwired: 14 in]
      }
      frame "UI: Update Lockin Graphs" {
        # "results"
        # "Do not put any code in this frame.\n(It is a separator no-op. You can make a copy of this frame to create a new UI frame)"
        n67 = Unbundle By Name(w202) -> ("Sweep Value"=w194:dbl, "Control Experiment"=w201:refnum<class "SMO.Control Experiment.lvclass">, "Results (Dictionary)"=w190:cluster{"key":string, "value":dbl}[])
        n68 = call "Get Channel Indices.vi"("Control Experiment in"=w201) -> ("Indices"=w200:T15)  [unwired: 8 in, 2 out]
        n69 = call <userlib>:"Parse Results (all).vi"("Type"=Results_Type--Enum."R", "error in (no error)"=w184, "Results (Dictionary)"=w190) -> ("error out"=w183:errorcluster, "Data"=w186:dbl[], "Results (Dictionary)"=w185:cluster{"key":string, "value":dbl}[])  [unwired: 5 in, 1 out]
        n70 = Unbundle By Name(w200) -> ("I-"=w197:i32, "V1+"=w199:i32, "V1-"=w198:i32)
        n71 = Less?(x=w193, y=20) -> (x < y?=w191:bool)
        n72 = call <userlib>:"Parse Results (all).vi"("Type"=Results_Type--Enum."Theta", "error in (no error)"=w183, "Results (Dictionary)"=w185) -> ("error out"=w182:errorcluster, "Data"=w187:dbl[])  [unwired: 5 in, 2 out]
        n73 = call "GraphLockin_vs_Parameter.vi"("V-"=w198, "V+"=w199, "reset?"=w191, "Current"=w197, "Parameter"=w194, "Y[ ]"=w187, "X[ ]"=w186) -> ("G(e2/h) vs Parameter"=→"G4T":cluster{"Y":dbl[], "Y":dbl[]}[], "Y vs Parameter"=→"Y Lockins":cluster{dbl[], dbl[]}[], "X vs Parameter"=→"X Lockins":cluster{dbl[], dbl[]}[])  [unwired: 1 in, 1 out]
        n74 = call <vilib>:"Add State(s) to Queue__jki_lib_state_machine.vi"("State(s) in (\"\")"=w205) -> ("States Out"=w204:string)  [unwired: 14 in]
      }
      frame "UI: Update Timer" {
        n75 = Unbundle By Name(w213) -> ("ms [0]"=w214:u32)
        n76 = call <userlib>:"Tick Count (ms)__ogtk.vi"("error in (no error)"=w215) -> ("error out"=w208:errorcluster, "millisecond timer value"=w206:u32)  [unwired: 9 in]
        n77 = Subtract(x=w206, y=w214) -> (x-y=w210:u32)
        n78 = call <userlib>:"MGI Milliseconds Since Last Call.vi"("Error In"=w208) -> ("ms"=→"time b/w points (ms)":u32, "Error Out"=w207:errorcluster)  [unwired: 5 in]
        n79 = Divide(x=w210, y=u32 1000 ("x")) -> (x/y=→"elapsed time (s)":dbl)
        n80 = Bundle By Name(cluster=w213, "ms [i]"=w206) -> (w212:T12)
        n81 = call <vilib>:"Add State(s) to Queue__jki_lib_state_machine.vi"("State(s) in (\"\")"=w218) -> ("States Out"=w217:string)  [unwired: 14 in]
      }
      frame "UI: Update Input Graphs" {
        # "AI and AO waveforms once the sweep completes"
        # "Do not put any code in this frame.\n(It is a separator no-op. You can make a copy of this frame to create a new UI frame)"
        n82 = Unbundle By Name(w222) -> ("Instruments.Lockin"=w223:refnum<class "Instrument.Lockin.lvclass">)
        n83 = call <userlib>:"getSweepWaveforms.vi"("Instrument.Lockin in"=w223) -> ("Sweep_AI"=w219:waveform(dbl)[], "Sweep_AO"=w220:waveform(dbl)[])  [unwired: 7 in, 2 out]
        n84 = call-poly <userlib>:"Index Array Elements__ogtk.vi"("indices"="AO indices", "array"=w220) -> ("elements"=w228:variant[])  [unwired: 9 in]
        n85 = Variant To Data(type=w220, Variant=w228) -> (data=→"AO Waveform":waveform(dbl)[])  [unwired: 1 in, 1 out]
        n86 = call-poly <userlib>:"Index Array Elements__ogtk.vi"("indices"="AI indices", "array"=w219) -> ("elements"=w229:variant[])  [unwired: 9 in]
        n87 = Variant To Data(type=w219, Variant=w229) -> (data=→"AI Waveform":waveform(dbl)[])  [unwired: 1 in, 1 out]
        n88 = Bundle By Name(cluster=w222, "Sweep_AO"=w220, "Sweep_AI"=w219) -> (w221:T12)
        n89 = call <vilib>:"Add State(s) to Queue__jki_lib_state_machine.vi"("State(s) in (\"\")"=w232) -> ("States Out"=w231:string)  [unwired: 14 in]
      }
      frame "UI: Update IV Graphs" {
        # "Do not put any code in this frame.\n(It is a separator no-op. You can make a copy of this frame to create a new UI frame)"
        n90 = Unbundle By Name(w242) -> ("Sweep_AI"=w237:waveform(dbl)[], "Sweep_AO"=w236:waveform(dbl)[], "Control Experiment"=w246:refnum<class "SMO.Control Experiment.lvclass">)
        n91 = call "Get Channel Indices.vi"("error in (no error)"=w241, "Control Experiment in"=w246) -> ("error out"=w240:errorcluster, "Indices"=w243:T15)  [unwired: 7 in, 1 out]
        n92 = Unbundle By Name(w243) -> ("I-"=w248:i32, "V1+"=w244:i32, "V1-"=w245:i32, "I+"=w247:i32)
        n93 = Decrement(x=w247) -> (x-1=w259:i32)
        n94 = Decrement(x=w248) -> (x-1=w250:i32)
        n95 = Decrement(x=w244) -> (x-1=w258:i32)
        n96 = Decrement(x=w245) -> (x-1=w253:i32)
        n97 = Index Array(array=w236, index=w259) -> (element=w260:waveform(dbl))
        n98 = Index Array(array=w237, index #1=w250, index #2=w258, index #3=w253) -> (element #1=w255:waveform(dbl), element #2=w252:waveform(dbl), element #3=w257:waveform(dbl))
        n99 = Equal?(x=w258, y=w253) -> (x = y?=w254:bool)
        n100 = Subtract(1:w257, 2:w252) -> (0:w251:waveform(dbl))  [unwired: 1 in, 1 out]
        n101 = Unbundle By Name(w260) -> ("Y"=w233:dbl[])
        n102 = Select(t=w252, s=w254, f=w251) -> (s? t:f=w256:waveform(dbl))
        n103 = Unbundle By Name(w255) -> ("Y"=w235:dbl[])
        n104 = Unbundle By Name(w256) -> ("Y"=w234:dbl[])
        n105 = Bundle("Y"=w234, "Y"=w235) -> (w249:cluster{"Y":dbl[], "Y":dbl[]})  [unwired: 1 in]
        n106 = Bundle("Y"=w233, "Y"=w235) -> (w261:cluster{"Y":dbl[], "Y":dbl[]})  [unwired: 1 in]
        n107 = Build Array(w249) -> (→"4Term":cluster{"Y":dbl[], "Y":dbl[]}[])
        n108 = Build Array(w261) -> (→"2Term":cluster{"Y":dbl[], "Y":dbl[]}[])
        n109 = call <vilib>:"Add State(s) to Queue__jki_lib_state_machine.vi"("State(s) in (\"\")"=w263) -> ("States Out"=w262:string)  [unwired: 14 in]
      }
      frame "UI: Front Panel State" {
        # "Argument"
        # "Set Front Panel Open or Closed\n(Usage: \"UI: Front Panel State >> Open|Close\")"
        n110 = Unbundle By Name(w266) -> ("Core.Current VI Reference"=w265:refnum<vi>)
        n111 = case shown="\"Minimize\", \"Minimized\"" w264 {
          tunnel: w268 -> [w276 w291 w302 w315 w328]
          tunnel: [w278 w292 w304 w317 w330] -> w267
          tunnel: w265 -> [w277 w289 w303 w316 w329]
          frame "Open", "Standard", Default {
            w271 = T7."Standard" ("State")
            n112 = property class="VI"(reference=w277, error in=w276) -> (reference out=w274:refnum<vi>, error out=w275:errorcluster, "FP.State"=w273:T7)
            n113 = Not Equal?(x=w273, y=w271) -> (x != y?=w272:bool)
            n114 = case shown="True" w272 {
              tunnel: [w282 w284] -> w278
              tunnel: w275 -> [w281 w284]
              tunnel: w274 -> [w280 _]
              tunnel: w271 -> [w279 _]
              frame True {
                n115 = invoke class="VI" method="FP.Open"(reference=w280, error in=w281, "Activate"=TRUE, "State"=w279) -> (error out=w282:errorcluster)  [unwired: 1 in, 4 out]
              }
              frame False {
              }
            }
          }
          frame "Close", "Closed" {
            n116 = property class="VI"(reference=w289, error in=w291) -> (reference out=w288:refnum<vi>, error out=w290:errorcluster, "FP.State"=w286:T7)
            n117 = Not Equal?(x=w286, y=T7."Closed" ("Front Panel Window:State")) -> (x != y?=w285:bool)
            n118 = case shown="True" w285 {
              tunnel: [w293 w296] -> w292
              tunnel: w290 -> [w293 w295]
              tunnel: w288 -> [_ w294]
              frame False {
              }
              frame True {
                n119 = invoke class="VI" method="FP.Close"(reference=w294, error in=w295) -> (error out=w296:errorcluster)  [unwired: 1 in, 2 out]
              }
            }
          }
          frame "Hidden", "Hide" {
            w297 = T7."Hidden" ("State")
            n120 = property class="VI"(reference=w303, error in=w302) -> (reference out=w300:refnum<vi>, error out=w301:errorcluster, "FP.State"=w299:T7)
            n121 = Not Equal?(x=w299, y=w297) -> (x != y?=w298:bool)
            n122 = case shown="True" w298 {
              tunnel: [w308 w309] -> w304
              tunnel: w301 -> [w307 w309]
              tunnel: w300 -> [w306 _]
              tunnel: w297 -> [w305 _]
              frame True {
                n123 = invoke class="VI" method="FP.Open"(reference=w306, error in=w307, "State"=w305) -> (error out=w308:errorcluster)  [unwired: 2 in, 4 out]
              }
              frame False {
              }
            }
          }
          frame "Minimize", "Minimized" {
            w310 = T7."Minimized" ("State")
            n124 = property class="VI"(reference=w316, error in=w315) -> (reference out=w313:refnum<vi>, error out=w314:errorcluster, "FP.State"=w312:T7)
            n125 = Not Equal?(x=w312, y=w310) -> (x != y?=w311:bool)
            n126 = case shown="True" w311 {
              tunnel: [w321 w322] -> w317
              tunnel: w314 -> [w320 w322]
              tunnel: w313 -> [w319 _]
              tunnel: w310 -> [w318 _]
              frame True {
                n127 = invoke class="VI" method="FP.Open"(reference=w319, error in=w320, "State"=w318) -> (error out=w321:errorcluster)  [unwired: 2 in, 4 out]
              }
              frame False {
              }
            }
          }
          frame "Maximize", "Maximized" {
            w323 = T7."Maximized" ("State")
            n128 = property class="VI"(reference=w329, error in=w328) -> (reference out=w326:refnum<vi>, error out=w327:errorcluster, "FP.State"=w325:T7)
            n129 = Not Equal?(x=w325, y=w323) -> (x != y?=w324:bool)
            n130 = case shown="True" w324 {
              tunnel: [w334 w335] -> w330
              tunnel: w327 -> [w333 w335]
              tunnel: w326 -> [w332 _]
              tunnel: w323 -> [w331 _]
              frame True {
                n131 = invoke class="VI" method="FP.Open"(reference=w332, error in=w333, "State"=w331) -> (error out=w334:errorcluster)  [unwired: 2 in, 4 out]
              }
              frame False {
              }
            }
          }
        }
        n132 = call <vilib>:"Add State(s) to Queue__jki_lib_state_machine.vi"("State(s) in (\"\")"=w270) -> ("States Out"=w269:string)  [unwired: 14 in]
      }
      frame "---------- Macro ----------" {
        # "Do not put any code in this frame.\n(It is a separator no-op. You can make a copy of this frame to create a new Macro frame)"
        n133 = call <vilib>:"Add State(s) to Queue__jki_lib_state_machine.vi"("State(s) in (\"\")"=w339) -> ("States Out"=w338:string)  [unwired: 14 in]
      }
      frame "Macro: Initialize" {
        # "Initialization Macro\n(This is called once, when the VI starts)"
        n134 = call <vilib>:"Add State(s) to Queue__jki_lib_state_machine.vi"("State(s) in Front (\"\")"="Data: Initialize\nInitialize Core Data\nUI: Initialize\nUI: Front Panel State >> Open\nData: Initialize Top Level\nSweep: Initialize\nMeasure: Temperature\nMeasure: Magnet\nMeasure: Capacitance\nSweep: Start", "State(s) in (\"\")"=w344) -> ("States Out"=w343:string)  [unwired: 13 in]
      }
      frame "Macro: Sweep" {
        # "Template Separator\n(You can make a copy of, or modify, this frame)"
        n135 = call <vilib>:"Add State(s) to Queue__jki_lib_state_machine.vi"("State(s) in Front (\"\")"="Measure: Time\nMeasure: Lockin\nUI: Update Lockin Graphs\nUI: Update Timer" ("State(s) in Front (\"\")"), "State(s) in (\"\")"=w349) -> ("States Out"=w348:string)  [unwired: 13 in]
      }
      frame "Macro: Exit" {
        # "Exit Macro\n(This is called once, when the VI exits)"
        n136 = Unbundle By Name(w356) -> ("Core.Close Panel on Exit?"=w355:bool)
        n137 = Select(t="UI: Front Panel State >> Close", s=w355, f="") -> (s? t:f=w352:string)
        n138 = call <vilib>:"Add State(s) to Queue__jki_lib_state_machine.vi"("State(s) in (\"\")"=w352, "State(s) at Back (\"\")"="Sweep: Stop\nFile: Save Lockin\nData: Cleanup\nExit") -> ("States Out"=w350:string)  [unwired: 13 in]
        n139 = call <vilib>:"Add State(s) to Queue__jki_lib_state_machine.vi"("State(s) in Front (\"\")"=w350, "State(s) in (\"\")"=w359) -> ("States Out"=w358:string)  [unwired: 13 in]
      }
      frame "---------- Sweep ----------" {
        # "Do not put any code in this frame.\n(It is a separator no-op. You can make a copy of this frame to create a new Macro frame)"
        n140 = call <vilib>:"Add State(s) to Queue__jki_lib_state_machine.vi"("State(s) in (\"\")"=w363) -> ("States Out"=w362:string)  [unwired: 14 in]
      }
      frame "Sweep: Initialize" {
        # "Do not put any code in this frame.\n(It is a separator no-op. You can make a copy of this frame to create a new Macro frame)"
        n141 = Unbundle By Name(w365) -> ("Instruments.Lockin"=w368:refnum<class "Instrument.Lockin.lvclass">)
        n142 = call <userlib>:"setSweepConfiguration.vi"("error in (no error)"=w367, "Configure Sweep"="Configure Sweep", "Instrument.Lockin in"=w368) -> ("error out"=w366:errorcluster)  [unwired: 7 in, 1 out]
        n143 = call <vilib>:"Add State(s) to Queue__jki_lib_state_machine.vi"("State(s) in (\"\")"=w370) -> ("States Out"=w369:string)  [unwired: 14 in]
      }
      frame "Sweep: Start" {
        # "wait for sweeping to start"
        # "Do not put any code in this frame.\n(It is a separator no-op. You can make a copy of this frame to create a new Macro frame)"
        n144 = Unbundle By Name(w376) -> ("Instruments.Lockin"=w375:refnum<class "Instrument.Lockin.lvclass">)
        n145 = call <userlib>:"startSweep.vi"("error in (no error)"=w374, "Instrument.Lockin in"=w375) -> ("error out"=w372:errorcluster, "Instrument.Lockin out"=w373:refnum<class "Instrument.Lockin.lvclass">)  [unwired: 8 in]
        n146 = while {
          shift-right: [w386] -> w371
          shift-left: w372 -> [w387]
          tunnel: w373 -> [w383]
          tunnel: [w382] -> _
          stop <- w384 stop-if-true
          n147 = call <userlib>:"Wait (ms)__ogtk.vi"("error in (no error)"=w387, "milliseconds to wait"=u32 1000) -> ("error out"=w381:errorcluster)  [unwired: 8 in, 1 out]
          n148 = call <userlib>:"getStatus.vi"("error in (no error)"=w381, "Instrument.Lockin"=w383) -> ("error out"=w386:errorcluster, "Status"=w385:T16, "Instrument.Lockin"=w382:refnum<class "Instrument.Lockin.lvclass">)  [unwired: 7 in]
          n149 = Equal?(x=State-enum."sweeping" ("Status"), y=w385) -> (x = y?=w384:bool)
        }
        n150 = call <vilib>:"Add State(s) to Queue__jki_lib_state_machine.vi"("State(s) in (\"\")"=w378) -> ("States Out"=w377:string)  [unwired: 14 in]
      }
      frame "Sweep: Stop" {
        # "Do not put any code in this frame.\n(It is a separator no-op. You can make a copy of this frame to create a new Macro frame)"
        n151 = Unbundle By Name(w391) -> ("Instruments.Lockin"=w390:refnum<class "Instrument.Lockin.lvclass">)
        n152 = call <userlib>:"stopSweep.vi"("error in (no error)"=w389, "Instrument.Lockin in"=w390) -> ("error out"=w388:errorcluster)  [unwired: 8 in, 1 out]
        n153 = call <vilib>:"Add State(s) to Queue__jki_lib_state_machine.vi"("State(s) in (\"\")"=w393) -> ("States Out"=w392:string)  [unwired: 14 in]
      }
      frame "Sweep: Check State" {
        # "Do not put any code in this frame.\n(It is a separator no-op. You can make a copy of this frame to create a new Macro frame)"
        n154 = Unbundle By Name(w399) -> ("Instruments.Lockin"=w398:refnum<class "Instrument.Lockin.lvclass">)
        n155 = call <userlib>:"getStatus.vi"("error in (no error)"=w397, "Instrument.Lockin"=w398) -> ("error out"=w396:errorcluster, "Status"=w395:T16)  [unwired: 7 in, 1 out]
        n156 = case shown="Default" w395 {
          tunnel: ["UI: Update Input Graphs\nUI: Update IV Graphs\nMacro: Exit" ("State(s) in Front (\"\")") "Macro: Sweep" ("State(s) in Front (\"\")")] -> w394
          frame Default {
          }
          frame "sweeping" {
          }
        }
        n157 = call <vilib>:"Add State(s) to Queue__jki_lib_state_machine.vi"("State(s) in Front (\"\")"=w394, "State(s) in (\"\")"=w401) -> ("States Out"=w400:string)  [unwired: 13 in]
      }
      frame "---------- Configure ----------" {
        # "Do not put any code in this frame.\n(It is a separator no-op. You can make a copy of this frame to create a new Macro frame)"
        n158 = call <vilib>:"Add State(s) to Queue__jki_lib_state_machine.vi"("State(s) in (\"\")"=w407) -> ("States Out"=w406:string)  [unwired: 14 in]
      }
      frame "Configure: Wait" {
        # "Do not put any code in this frame.\n(It is a separator no-op. You can make a copy of this frame to create a new Macro frame)"
        n159 = call <vilib>:"Add State(s) to Queue__jki_lib_state_machine.vi"("State(s) in (\"\")"=w411) -> ("States Out"=w410:string)  [unwired: 14 in]
      }
      frame "---------- Measure ----------" {
        # "Template Separator\n(You can make a copy of, or modify, this frame)"
        n160 = call <vilib>:"Add State(s) to Queue__jki_lib_state_machine.vi"("State(s) in (\"\")"=w415) -> ("States Out"=w414:string)  [unwired: 14 in]
      }
      frame "Measure: Time" {
        # "Your code here.\n(You can make a copy of, or modify, this frame)"
        n161 = Unbundle By Name(w422) -> ("Control Experiment"=w420:refnum<class "SMO.Control Experiment.lvclass">)
        n162 = Get Date/Time In Seconds() -> (seconds since 1Jan1904=w424:timestamp)
        n163 = To Double Precision Float(number=w424) -> (double precision float=w418:dbl)
        n164 = call "Write Dictionary Element.vi"("error in (no error)"=w417, "value"=w418, "key"="Time", "Control Experiment in"=w420) -> ("error out"=w416:errorcluster, "Control Experiment out"=w421:refnum<class "Control Experiment.lvclass">)  [unwired: 6 in]
        n165 = Bundle By Name(cluster=w422, "Time"=w418, "Control Experiment"=w421) -> (w423:T12)
        n166 = call <vilib>:"Add State(s) to Queue__jki_lib_state_machine.vi"("State(s) in (\"\")"=w426) -> ("States Out"=w425:string)  [unwired: 14 in]
      }
      frame "Measure: Temperature" {
        # "Your code here.\n(You can make a copy of, or modify, this frame)"
        n167 = Unbundle By Name(w435) -> ("Control Experiment"=w429:refnum<class "SMO.Control Experiment.lvclass">, "Instruments.Temperature"=w437:refnum<class "Instrument.Cryostat.lvclass">)
        n168 = call-dynamic "Get Temperature.vi"("error in (no error)"=w436, "Instrument.Cryostat in"=w437) -> ("error out"=w431:errorcluster, "Temperature (K)"=w430:dbl, "Instrument.Cryostat out"=w427:refnum<class "Instrument.Cryostat.lvclass">)  [unwired: 5 in, 2 out]
        "T (mK)" <- w430
        n169 = call "Write Dictionary Element.vi"("error in (no error)"=w431, "value"=w430, "key"="Temperature", "Control Experiment in"=w429) -> ("error out"=w428:errorcluster, "Control Experiment out"=w433:refnum<class "Control Experiment.lvclass">)  [unwired: 6 in]
        n170 = Bundle By Name(cluster=w435, "Instruments.Temperature"=w427, "Control Experiment"=w433) -> (w434:T12)
        n171 = call <vilib>:"Add State(s) to Queue__jki_lib_state_machine.vi"("State(s) in (\"\")"=w439) -> ("States Out"=w438:string)  [unwired: 14 in]
      }
      frame "Measure: Magnet" {
        # "Your code here.\n(You can make a copy of, or modify, this frame)"
        n172 = Unbundle By Name(w450) -> ("Control Experiment"=w445:refnum<class "SMO.Control Experiment.lvclass">, "Instruments.Magnet"=w444:refnum<class "Instrument.Cryostat.lvclass">)
        n173 = call-dynamic "Get Magnet Field.vi"("error in (no error)"=w443, "Instrument.Cryostat in"=w444) -> ("error out"=w442:errorcluster, "B Field (T)"=w441:dbl, "Instrument.Cryostat out"=w440:refnum<class "Instrument.Cryostat.lvclass">)  [unwired: 5 in, 2 out]
        "Field (T)" <- w441
        n174 = call "Write Dictionary Element.vi"("error in (no error)"=w442, "value"=w441, "key"="Magnet", "Control Experiment in"=w445) -> ("error out"=w446:errorcluster, "Control Experiment out"=w448:refnum<class "Control Experiment.lvclass">)  [unwired: 6 in]
        n175 = Bundle By Name(cluster=w450, "Instruments.Magnet"=w440, "Control Experiment"=w448) -> (w449:T12)
        n176 = call <vilib>:"Add State(s) to Queue__jki_lib_state_machine.vi"("State(s) in (\"\")"=w452) -> ("States Out"=w451:string)  [unwired: 14 in]
      }
      frame "Measure: Capacitance" {
        # "Your code here.\n(You can make a copy of, or modify, this frame)"
        n177 = Unbundle By Name(w453) -> ("Control Experiment"=w458:refnum<class "SMO.Control Experiment.lvclass">, "Instruments.Level"=w456:refnum<class "Instrument.Cryostat.lvclass">)
        n178 = call-dynamic "Get Capacitance.vi"("error in (no error)"=w457, "Instrument.CBridge in"=w456) -> ("error out"=w454:errorcluster, "Capacitance (pF)"=w455:dbl)  [unwired: 7 in, 1 out]
        n179 = call "Write Dictionary Element.vi"("error in (no error)"=w454, "value"=w455, "key"="Capacitance", "Control Experiment in"=w458) -> ("error out"=w459:errorcluster, "Control Experiment out"=w461:refnum<class "Control Experiment.lvclass">)  [unwired: 6 in]
        n180 = Bundle By Name(cluster=w453, "Control Experiment"=w461) -> (w462:T12)
        n181 = call <vilib>:"Add State(s) to Queue__jki_lib_state_machine.vi"("State(s) in (\"\")"=w464) -> ("States Out"=w463:string)  [unwired: 14 in]
      }
      frame "Measure: Lockin" {
        # "Demodulated AI"
        # "Gives the AI and AO waveform which refreshes as per the Lockin sampling parameters"
        # "Template Separator\n(You can make a copy of, or modify, this frame)"
        n182 = local read "Configure Sweep"() -> (w469:T2)
        n183 = Unbundle By Name(w465) -> ("Instruments.Lockin"=w481:refnum<class "Instrument.Lockin.lvclass">)
        n184 = Unbundle By Name(w469) -> ("Channels"=w471:T3)
        n185 = Index Array(array=w471) -> (element=w468:T4)  [unwired: 1 in]
        n186 = Unbundle By Name(w468) -> ("Channel"=w467:u16)
        n187 = call <userlib>:"getAO.vi"("error in (no error)"=w482, "Instrument.Lockin in"=w481) -> ("error out"=w477:errorcluster, "AOconfig"=w475:T17, "Instrument.Lockin out"=w480:refnum<class "Instrument.Lockin.lvclass">)  [unwired: 7 in]
        n188 = Decrement(x=w467) -> (x-1=w470:u16)
        n189 = call <userlib>:"getAIwfm.vi"("error in (no error)"=w477, "Instrument.Lockin in"=w480) -> ("error out"=w476:errorcluster, "AI Waveform"=w478:waveform(dbl)[], "Instrument.Lockin out"=w479:refnum<class "Instrument.Lockin.lvclass">)  [unwired: 7 in]
        n190 = Index Array(array=w475, index=w470) -> (element=w474:T18)
        n191 = call <userlib>:"getResults.vi"("error in (no error)"=w476, "Instrument.Lockin in"=w479) -> ("error out"=w484:errorcluster, "Results (Dictionary)"=w483:cluster{"key":string, "value":dbl}[])  [unwired: 6 in, 2 out]
        n192 = Unbundle By Name(w474) -> ("Y"=w473)
        n193 = Index Array(array=w473) -> (element=w472)  [unwired: 1 in]
        n194 = Bundle By Name(cluster=w465, "AO Waveforrm"=w475, "AI Waveform"=w478, "Results (Dictionary)"=w483, "Sweep Value"=w472) -> (w466:T12)
        n195 = call <vilib>:"Add State(s) to Queue__jki_lib_state_machine.vi"("State(s) in (\"\")"=w486) -> ("States Out"=w485:string)  [unwired: 14 in]
      }
      frame "---------- File ----------" {
        # "Template Separator\n(You can make a copy of, or modify, this frame)"
        n196 = call <vilib>:"Add State(s) to Queue__jki_lib_state_machine.vi"("State(s) in (\"\")"=w490) -> ("States Out"=w489:string)  [unwired: 14 in]
      }
      frame "File: Configure" {
        # "Template Separator\n(You can make a copy of, or modify, this frame)"
        n197 = call <vilib>:"Add State(s) to Queue__jki_lib_state_machine.vi"("State(s) in (\"\")"=w494) -> ("States Out"=w493:string)  [unwired: 14 in]
      }
      frame "File: Save Lockin" {
        # "build wavename label"
        # "build cluster array(s) of multiple 1D data, dynamically name waves"
        # "build wavename array"
        # "Template Separator\n(You can make a copy of, or modify, this frame)"
        n198 = Unbundle By Name(w516) -> ("Control Experiment"=w525:refnum<class "SMO.Control Experiment.lvclass">, "Instruments.Lockin"=w514:refnum<class "Instrument.Lockin.lvclass">, "Execution:State"=w518:T13, "Sweep_AO"=w511:waveform(dbl)[], "Sweep_AI"=w509:waveform(dbl)[])
        n199 = call <userlib>:"getSweepResults.vi"("error in (no error)"=w498, "Instrument.Lockin in"=w514) -> ("error out"=w495:errorcluster, "Y Results"=w496:waveform(dbl)[], "X results"=w497:waveform(dbl)[])  [unwired: 6 in, 1 out]
        n200 = call "Waveform to Cluster.vi"("Input"=w511, "Input String"="AO") -> ("Output"=w499:cluster{"Y":dbl[]}[], "Output Label"=w506:string[])  [unwired: 7 in, 1 out]
        n201 = call "Waveform to Cluster.vi"("Input"=w496, "Input String"="Y") -> ("Output"=w502:cluster{"Y":dbl[]}[], "Output Label"=w503:string[])  [unwired: 7 in, 1 out]
        n202 = call "Waveform to Cluster.vi"("Input"=w509, "Input String"="AI") -> ("Output"=w500:cluster{"Y":dbl[]}[], "Output Label"=w505:string[])  [unwired: 7 in, 1 out]
        n203 = call "Waveform to Cluster.vi"("Input"=w497, "Input String"="X") -> ("Output"=w501:cluster{"Y":dbl[]}[], "Output Label"=w504:string[])  [unwired: 7 in, 1 out]
        n204 = call "Get Channel Indices.vi"("Control Experiment in"=w525) -> ("Control Experiment out"=w522:refnum<class "Control Experiment.lvclass">)  [unwired: 8 in, 2 out]
        n205 = Build Array (concatenate)(w506, w505, w504, w503) -> (w523:string[])
        n206 = Build Array (concatenate)(w499, w500, w501, w502) -> (w524:cluster{"Y":dbl[]}[])
        n207 = for {
          tunnel: w524 -> [w529] mode=indexing
          tunnel: w523 -> [w528] mode=indexing
          tunnel: [w531] -> w521
          tunnel: w495 -> [w530]
          shift-right: [w532] -> w520
          shift-left: w522 -> [w533]
          n208 = call "Write Dictionary Element.vi"("error in (no error)"=w530, "value"=w529, "key"=w528, "Control Experiment in"=w533) -> ("error out"=w531:errorcluster, "Control Experiment out"=w532:refnum<class "Control Experiment.lvclass">)  [unwired: 6 in]
        }
        n209 = call "Exec State to Append.vi"("Execution:State"=w518) -> ()  [unwired: 2 in, 1 out]
        n210 = call "Save Transport TDMS File.vi"("error in (no error)"=w521, 10:FALSE ("append?"), "Control Experiment in"=w520) -> ("error out"=w519:errorcluster, "Control Experiment out"=w517:refnum<class "Control Experiment.lvclass">)  [unwired: 7 in]
        n211 = Bundle By Name(cluster=w516, "Control Experiment"=w517) -> (w515:T12)
        n212 = call <vilib>:"Add State(s) to Queue__jki_lib_state_machine.vi"("State(s) in (\"\")"=w527) -> ("States Out"=w526:string)  [unwired: 14 in]
      }
      frame "File: JSON" {
        # "Template Separator\n(You can make a copy of, or modify, this frame)"
        n213 = local read "Configure Sweep"() -> (w538:T2)
        n214 = Unbundle By Name(w543) -> ("Control Experiment"=w540:refnum<class "SMO.Control Experiment.lvclass">)
        n215 = Unbundle By Name(w538) -> ("Sweep Time (s)"=w534:dbl, "Initial Wait (s)"=w535:dbl, "Return to Start"=w536:bool, "Channels"=w537:T3)
        n216 = Bundle By Name(cluster=T2 {"Sweep Time (s)"=0.0, "Initial Wait (s)"=0.0, "Return to Start"=FALSE, "Channels"=[]} ("Configure Sweep"), "Sweep Time (s)"=w534, "Initial Wait (s)"=w535, "Return to Start"=w536, "Channels"=w537) -> (w544:T2)
        n217 = call "Save JSON File.vi"("error in (no error)"=w542, "Data"=w544, "Control Experiment in"=w540) -> ("error out"=w541:errorcluster)  [unwired: 8 in]
        n218 = call <vilib>:"Add State(s) to Queue__jki_lib_state_machine.vi"("State(s) in (\"\")"=w546) -> ("States Out"=w545:string)  [unwired: 14 in]
      }
    }
  }
  "error out" <- w2
  n219 = Unbundle By Name(w4) -> ("Transport"=→"Transport out":refnum<class "SMO.Transport.lvclass">)
